vi "Clean_Up_Template.vi"(1 "Template Info In":string[](array[string])) -> (0 "Template Info Out":string[](array[string]))   [LabVIEW 2015]
uses:
  Controls/Global_mode.ctl
panel:
  in  "Mode":T1
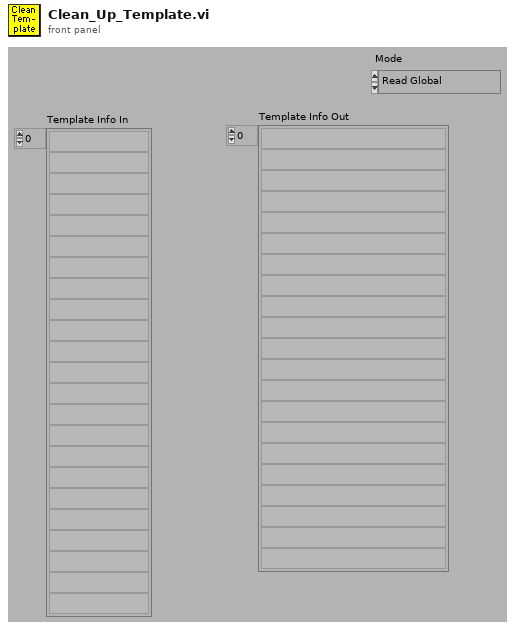
[diagram p1: front panel]
types:
  T1 = typedef "Global_mode.ctl" = enum16{"Read Global", "Load Global From File", "Write Global to File"}
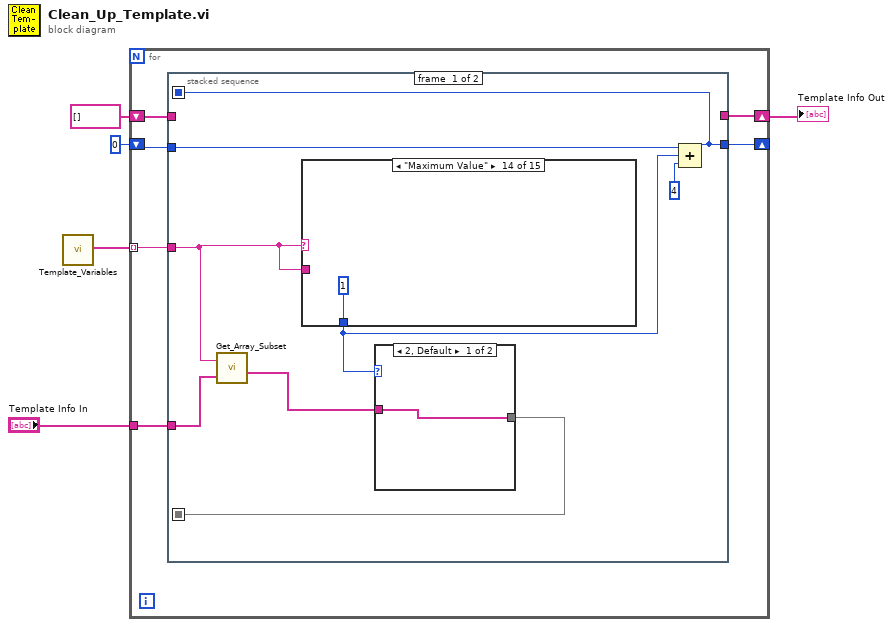
[diagram p0: block diagram]
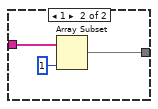
[diagram p2: hidden frame]
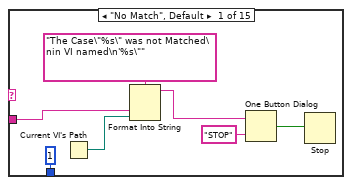
[diagram p3: hidden frame]
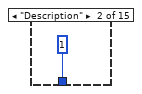
[diagram p4: hidden frame]
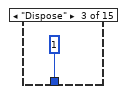
[diagram p5: hidden frame]
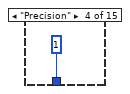
[diagram p6: hidden frame]
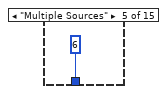
[diagram p7: hidden frame]
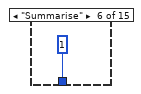
[diagram p8: hidden frame]
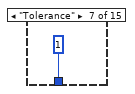
[diagram p9: hidden frame]
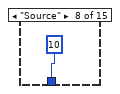
[diagram p10: hidden frame]
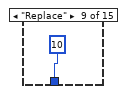
[diagram p11: hidden frame]
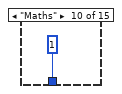
[diagram p12: hidden frame]
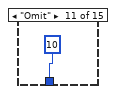
[diagram p13: hidden frame]
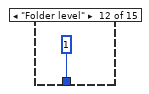
[diagram p14: hidden frame]
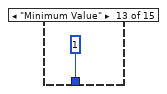
[diagram p15: hidden frame]
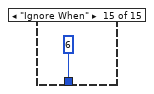
[diagram p16: hidden frame]
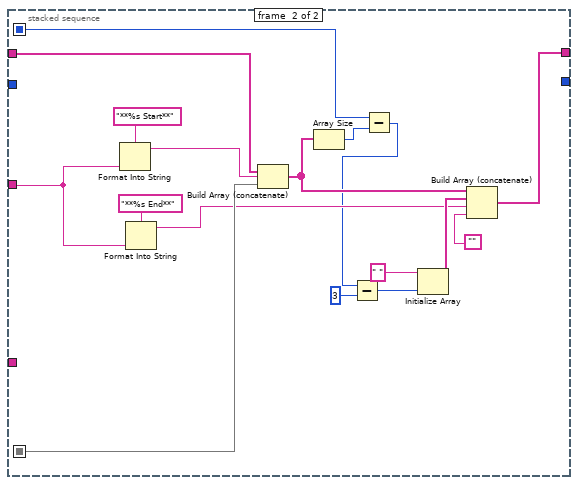
[diagram p17: hidden frame]
diagram:
  n1 = call "Template_Variables.vi"() -> ("Variable Names"=w1:string[])
  n2 = for {
    shift-right: [w6] -> w2
    shift-left: string[] [] -> [w7]
    tunnel: w1 -> [w11] mode=indexing
    tunnel: "Template Info In" -> [w10]
    shift-right: [w8] -> _
    shift-left: 0 -> [w9]
    n3 = stacked-sequence {
      seq-local: [w16 _] -> [_ w56]
      seq-local: [w12 _] -> [_ w54]
      tunnel: w11 -> [w18 w59]
      tunnel: w10 -> [w19 _]
      tunnel: w9 -> [w15 _]
      tunnel: [w12 _] -> w8
      tunnel: w7 -> [_ w58]
      tunnel: [_ w51] -> w6
      frame #0 {
        n4 = call "Get_Array_Subset.vi"("String Array In"=w19, "Subset Name"=w18) -> ("Array Subset Out"=w17:string[])  [unwired: 4 out]
        n5 = case shown="\"Maximum Value\"" w18 {
          tunnel: w18 -> [w25 _ _ _ _ _ _ _ _ _ _ _ _ _ _]
          tunnel: [1 1 1 1 6 1 1 10 10 1 10 1 1 1 6] -> w14
          frame "No Match", Default {
            n6 = Current VI's Path() -> (path=w26:path)
            n7 = Format Into String(format string="The Case\"%s\" was not Matched\nin VI named\n'%s\"" ("Format String"), w25, w26) -> (resulting string=w29:string)  [unwired: 2 in, 1 out]
            n8 = One Button Dialog(message=w29, button name ("OK")="STOP") -> (true=w27:bool)
            n9 = Stop(stop? (T)=w27) -> ()
          }
          frame "Description" {
          }
          frame "Dispose" {
          }
          frame "Precision" {
          }
          frame "Multiple Sources" {
          }
          frame "Summarise" {
          }
          frame "Tolerance" {
          }
          frame "Source" {
          }
          frame "Replace" {
          }
          frame "Maths" {
          }
          frame "Omit" {
          }
          frame "Folder level" {
          }
          frame "Minimum Value" {
          }
          frame "Maximum Value" {
          }
          frame "Ignore When" {
          }
        }
        n10 = case shown="2, Default" w14 {
          tunnel: w17 -> [w20 w23]
          tunnel: [w20 w22] -> w16
          frame 2, Default {
          }
          frame 1 {
            n11 = Array Subset(array=w23, length=1 ("Array Length")) -> (w22:string[])  [unwired: 1 in]
          }
        }
        n12 = Compound Arithmetic op=ADD(w15, w14, 4) -> (w12:i32)
      }
      frame #1 {
        n13 = Format Into String(format string="**%s Start**" ("Format String"), w59) -> (resulting string=w57:string)  [unwired: 2 in, 1 out]
        n14 = Format Into String(format string="**%s End**" ("Format String"), w59) -> (resulting string=w49:string)  [unwired: 2 in, 1 out]
        n15 = Build Array (concatenate)(w58, w57, w56) -> (w53:string[])
        n16 = Array Size(array=w53) -> (size(s)=w55:i32)
        n17 = Subtract(x=w54, y=w55) -> (x-y=w48:i32)
        n18 = Subtract(x=w48, y=3) -> (x-y=w50:i32)
        n19 = Initialize Array(" ", w50) -> (w52:string[])
        n20 = Build Array (concatenate)(w53, w52, w49, "") -> (w51:string[])
      }
    }
  }
  "Template Info Out" <- w2
